vi "Initial Values-Compare-DBL.vi"(5 "Function (Add)":T3=enum."Add", 7 "Current values":dbl[](array[numeric]), 8 "error in (no error)":errorcluster, 9 "Keys Array":T2, 10 "Section name":string, 11 "User profile ini file ref":T5) -> (0 "error out":errorcluster, 1 "Output info":T1, 2 "Changed parameters info":T4[](array[typedef]), 3 "User profile ini file ref":T5, 4 "Changes exist":bool)   [LabVIEW 2013]
uses:
  Typedefs/Ini file interface (DBL).ctl
  <vilib>/Utility/config.llb/Config Data RefNum.ctl
  User Interface/User profiles code/Typedefs/Changed parameter cluster.ctl
  User Interface/User profiles code/Typedefs/Comparison states.ctl
  User Interface/User profiles code/Typedefs/Changes info cluster-DBL.ctl
  Program Files (x86)/National Instruments/LabVIEW 2013/user.lib/_OpenG.lib/array/array.llb/Search 1D Array (Boolean)__ogtk.vi
  Program Files (x86)/National Instruments/LabVIEW 2013/user.lib/_OpenG.lib/array/array.llb/Index 1D Array Elements (DBL)__ogtk.vi
  Program Files (x86)/National Instruments/LabVIEW 2013/user.lib/_OpenG.lib/array/array.llb/Index 1D Array Elements (Variant)__ogtk.vi
  <vilib>/Utility/config.llb/NI_LVConfig.lvlib
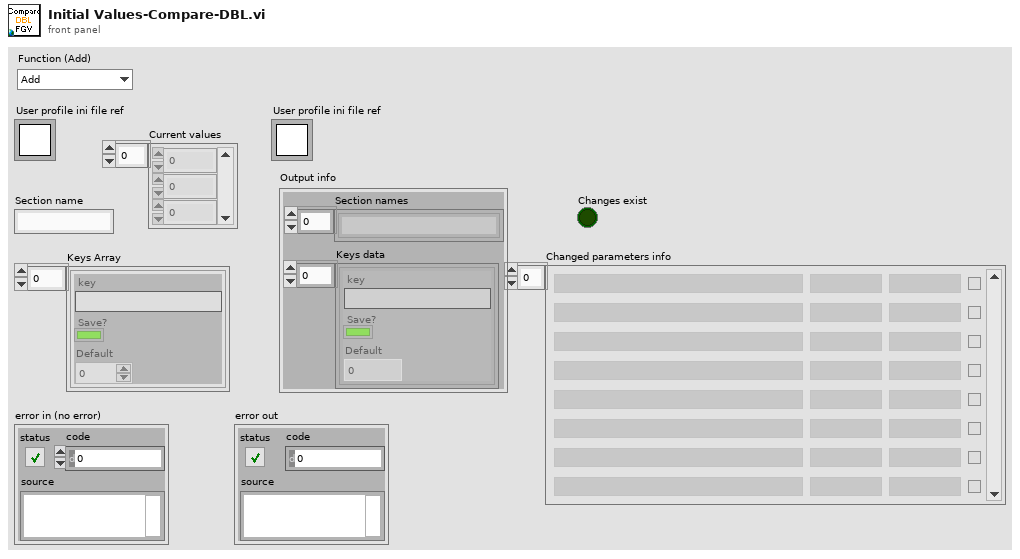
[diagram p1: front panel]
types:
  T1 = typedef "Changes info cluster-DBL.ctl" = cluster{"Section names":string[], "Keys data":T2}
  T2 = typedef "Ini file interface (DBL).ctl" = cluster{"key":string, "Save?":bool, "Default":dbl}[]
  T3 = typedef "Comparison states.ctl" = enum16{"Init.", "Add", "Read"}
  T4 = typedef "Changed parameter cluster.ctl" = cluster{"Name":string, "Old value":string, "New value":string, "Save":bool}
  T5 = typedef "NI_LVConfig.lvlib/Config Data RefNum.ctl" = refnum<k1>
  T6 = cluster{"key":string, "Save?":bool, "Default":dbl}
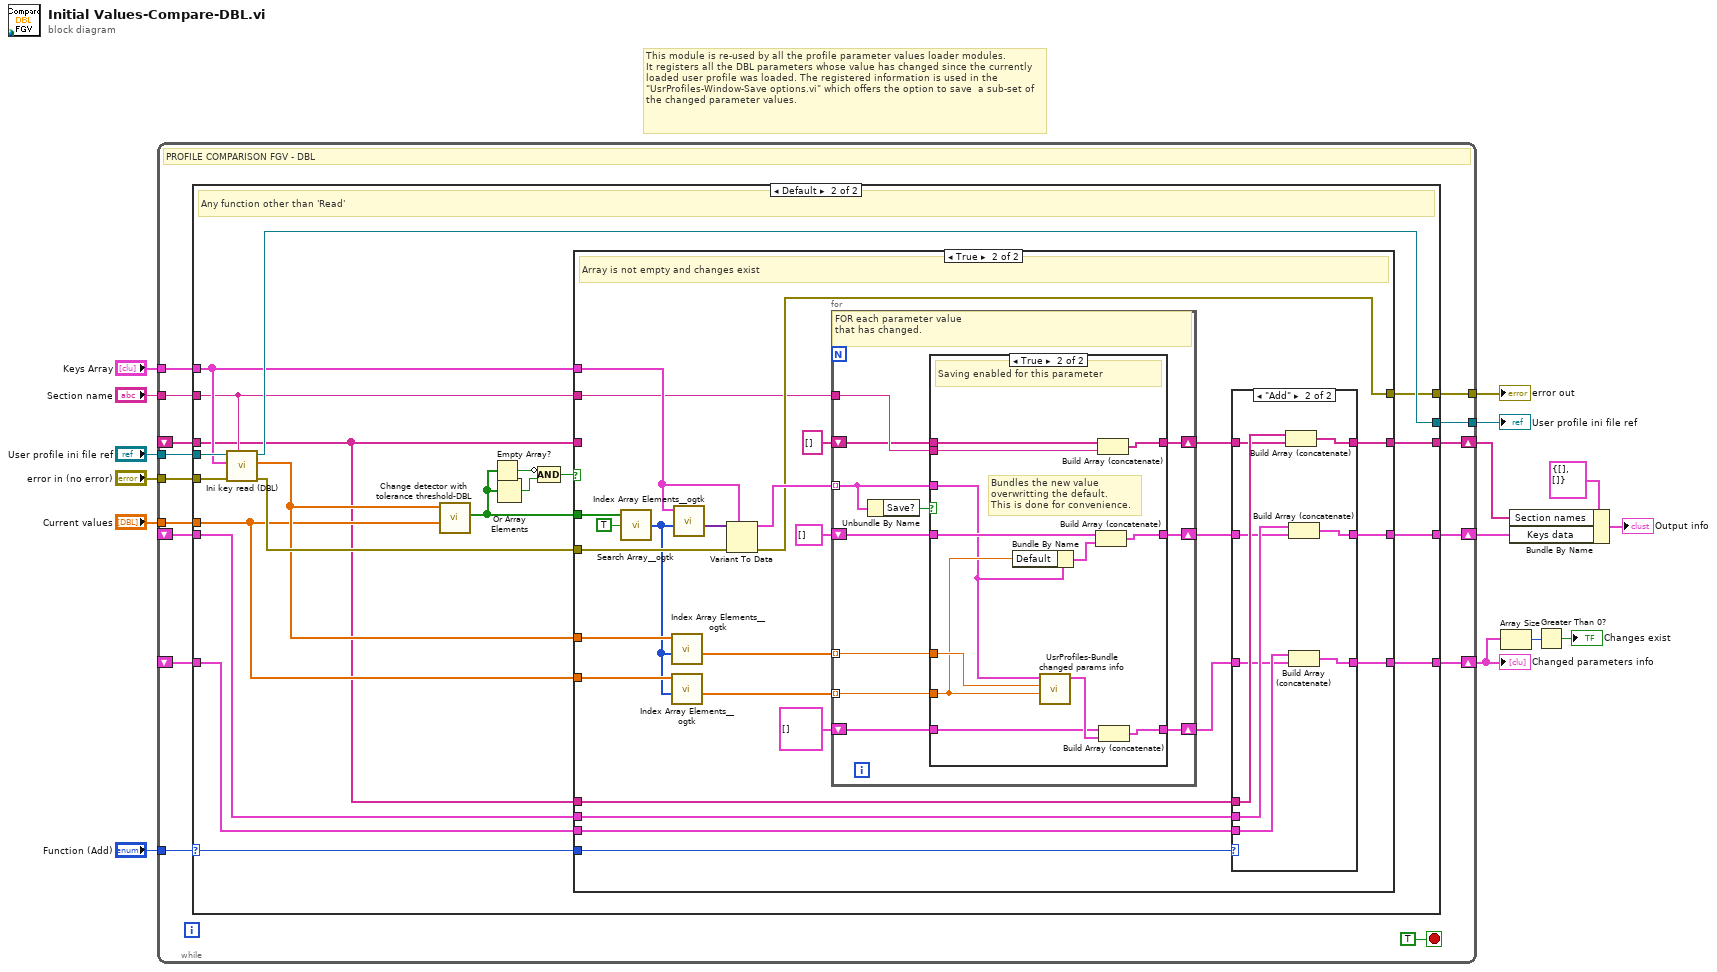
[diagram p0: block diagram]
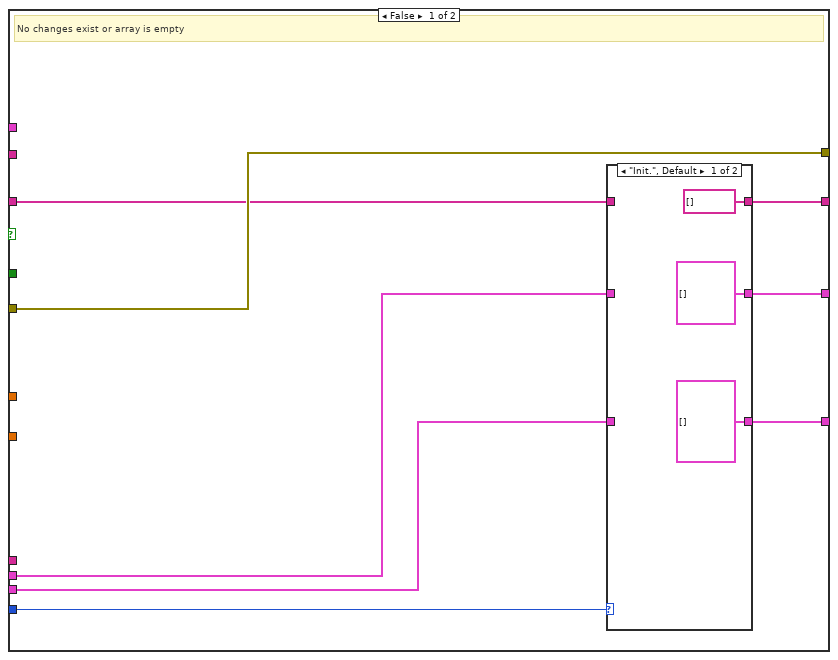
[diagram p3: hidden frame]
diagram:
  # "This module is re-used by all the profile parameter values loader modules.\nIt registers all the DBL parameters whose value has changed since the currently loaded user profile was loaded. The registered information is used in the \"UsrProfiles-Window-Save options.vi\" which offers the option to save  a sub-set of the changed parameter values."
  n1 = while {
    tunnel: "Section name" -> [w30]
    tunnel: "error in (no error)" -> [w29]
    tunnel: [w28] -> w13
    tunnel: "User profile ini file ref" -> [w27]
    tunnel: "Keys Array" -> [w26]
    tunnel: "Current values" -> [w20]
    tunnel: [w24] -> w9
    shift-right: [w19] -> w3
    shift-left: _ -> [w22]
    shift-right: [w23] -> w7
    shift-left: _ -> [w21]
    tunnel: "Function (Add)" -> [w18]
    shift-right: [w17] -> w4
    shift-left: _ -> [w16]
    stop <- TRUE stop-if-true
    # "PROFILE COMPARISON FGV - DBL"
    n2 = case shown="Default" w18 {
      selector: w18 -> [_ w39]
      tunnel: w30 -> [_ w38]
      tunnel: w29 -> [w35 w55]
      tunnel: [w34 w54] -> w28
      tunnel: w27 -> [w34 w53]
      tunnel: w26 -> [_ w52]
      tunnel: [w35 w50] -> w24
      tunnel: [w32 w49] -> w23
      tunnel: w22 -> [w33 w48]
      tunnel: w21 -> [w32 w47]
      tunnel: w20 -> [_ w42]
      tunnel: [w33 w40] -> w19
      tunnel: [w31 w37] -> w17
      tunnel: w16 -> [w31 w36]
      frame "Read" {
        # "The selected function is 'Read'"
      }
      frame Default {
        # "Any function other than 'Read'"
        n3 = call "Ini key read (DBL).vi"("Section name"=w38, "error in (no error)"=w55, "Parameter names & setup"=w52, "Ini file refnum in"=w53) -> ("error out"=w51:errorcluster, "Value read/used"=w43:dbl[], "Ini file refnum out"=w54:T5)  [unwired: 5 in]
        n4 = call "Change detector with tolerance threshold-DBL.vi"("From file"=w42, "Current values"=w43) -> ("Changed?"=w41:bool[])  [unwired: 9 in]
        n5 = Empty Array?(array=w41) -> (empty?=w46:bool)
        n6 = Or Array Elements(Boolean array=w41) -> (logical OR=w45:bool)
        n7 = Compound Arithmetic op=AND(invert w46, w45) -> (w44:bool)
        n8 = case shown="True" w44 {
          tunnel: w52 -> [_ w95]
          tunnel: w42 -> [_ w94]
          tunnel: w41 -> [_ w93]
          tunnel: w51 -> [w63 w90]
          tunnel: w43 -> [_ w89]
          tunnel: w39 -> [w58 w84]
          tunnel: [w63 w78] -> w50
          tunnel: [w59 w81] -> w49
          tunnel: w48 -> [w62 w80]
          tunnel: w47 -> [w61 w79]
          tunnel: [w60 w76] -> w40
          tunnel: w38 -> [_ w75]
          tunnel: [w56 w72] -> w37
          tunnel: w36 -> [w57 _]
          tunnel: w36 -> [_ w71]
          frame False {
            # "No changes exist or array is empty"
            n9 = case shown="\"Init.\", Default" w58 {
              tunnel: w62 -> [_ w68]
              tunnel: w61 -> [_ w69]
              tunnel: [T4[] [] w69] -> w59
              tunnel: [T2 [] ("Keys data") w68] -> w60
              tunnel: w57 -> [_ w67]
              tunnel: [string[] [] w67] -> w56
              frame "Init.", Default {
              }
              frame "Add" {
              }
            }
          }
          frame True {
            # "Array is not empty and changes exist"
            n10 = call-poly "Search Array__ogtk.vi"("Array"=w93, "Element Data"=TRUE) -> ("Indices of Elements"=w87:i32[])  [unwired: 7 in]
            n11 = call-poly "Index Array Elements__ogtk.vi"("indices"=w87, "array"=w89) -> ("elements"=w88:dbl[])  [unwired: 9 in]
            n12 = call-poly "Index Array Elements__ogtk.vi"("indices"=w87, "array"=w94) -> ("elements"=w86:dbl[])  [unwired: 9 in]
            n13 = call-poly "Index Array Elements__ogtk.vi"("indices"=w87, "array"=w95) -> ("elements"=w91:variant[])  [unwired: 9 in]
            n14 = Variant To Data(error in=w90, type=w95, Variant=w91) -> (data=w85:T2, error out=w78:errorcluster)
            n15 = for {
              tunnel: w88 -> [w118] mode=indexing
              tunnel: w86 -> [w117] mode=indexing
              tunnel: w85 -> [w114] mode=indexing
              shift-right: [w115] -> w83
              shift-left: T2 [] ("Keys data") -> [w116]
              shift-right: [w113] -> w82
              shift-left: T4[] [] -> [w112]
              tunnel: w75 -> [w110]
              shift-right: [w109] -> w73
              shift-left: string[] [] -> [w108]
              # "FOR each parameter value\nthat has changed."
              n16 = Unbundle By Name(w114) -> ("Save?"=w111:bool)
              n17 = case shown="True" w111 {
                tunnel: w118 -> [_ w133]
                tunnel: w117 -> [_ w132]
                tunnel: w116 -> [w121 w131]
                tunnel: [w121 w129] -> w115
                tunnel: w114 -> [_ w122]
                tunnel: [w120 w127] -> w113
                tunnel: w112 -> [w120 w126]
                tunnel: w110 -> [_ w123]
                tunnel: [w119 w125] -> w109
                tunnel: w108 -> [w119 w124]
                frame False {
                  # "Saving disabled for this parameter"
                }
                frame True {
                  # "Bundles the new value\noverwritting the default.\nThis is done for convenience."
                  # "Saving enabled for this parameter"
                  n18 = Bundle By Name(cluster=w122, "Default"=w132) -> (w130:T6)
                  n19 = call "UsrProfiles-Bundle changed params info.vi"("Current value"=w132, "Saved value"=w133, "Cluster in"=w122) -> ("Cluster out"=w128:T4)  [unwired: 8 in]
                  n20 = Build Array (concatenate)(w131, w130) -> (w129:T2)
                  n21 = Build Array (concatenate)(w124, w123) -> (w125:string[])
                  n22 = Build Array (concatenate)(w126, w128) -> (w127:T4[])
                }
              }
            }
            n23 = case shown="\"Add\"" w84 {
              tunnel: w83 -> [w97 w100]
              tunnel: w82 -> [w98 w99]
              tunnel: [w98 w107] -> w81
              tunnel: w80 -> [_ w103]
              tunnel: w79 -> [_ w104]
              tunnel: [w97 w106] -> w76
              tunnel: w73 -> [w96 w101]
              tunnel: [w96 w105] -> w72
              tunnel: w71 -> [_ w102]
              frame "Init.", Default {
              }
              frame "Add" {
                n24 = Build Array (concatenate)(w102, w101) -> (w105:string[])
                n25 = Build Array (concatenate)(w103, w100) -> (w106:T2)
                n26 = Build Array (concatenate)(w104, w99) -> (w107:T4[])
              }
            }
          }
        }
      }
    }
  }
  "User profile ini file ref" <- w13
  "error out" <- w9
  "Changed parameters info" <- w7
  n27 = Array Size(array=w7) -> (size(s)=w6:i32)
  n28 = Bundle By Name(cluster=T1 {"Section names"=[], "Keys data"=[]} ("Output info"), "Section names"=w4, "Keys data"=w3) -> (→"Output info":T1)
  n29 = Greater Than 0?(x=w6) -> (x > 0?=→"Changes exist":bool)
